vi "Same name VI.vi"(8 "Numeric":dbl=4.0) -> (0 "Numeric 2":dbl)   [LabVIEW 2023, in "Library.lvlib"]
uses:
  Library.lvlib
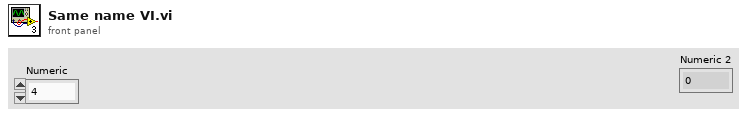
[diagram p1: front panel]
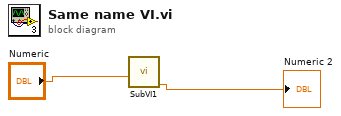
[diagram p0: block diagram]
diagram:
  n1 = call "SubVI1.vi"("x"="Numeric") -> ("x+y"=→"Numeric 2":dbl)  [unwired: 10 in]
